vi "Stop Core.vi"(10 "final error code":i32, 11 "Red Pitaya in":refnum<class "Red Pitaya.lvclass">) -> (3 "Red Pitaya out":refnum<class "Red Pitaya.lvclass">)   [LabVIEW 2015, in "Red Pitaya.lvclass"]
doc: "(<B>Filename</B>: Actor Framework.lvlib:Actor.lvclass:Stop Core.vi)\n\nDefines what the actor does before it stops. Use the <B>final error code</B> input to determine whether the actor shut down in response to an error.\n\nBy default, this method does nothing. A descendant class may override it to define behavior, such as shutting down any processes the actor initiated in its override of the Actor Core method."
uses:
  Red Pitaya.lvclass
  Mag Lab Measure/Hardware/Digitizer/Mag Lab Digitizer.lvclass
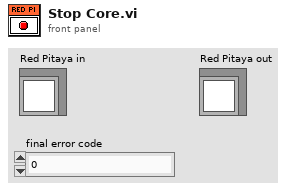
[diagram p1: front panel]
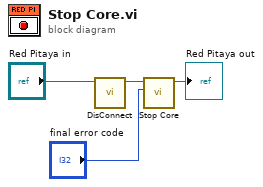
[diagram p0: block diagram]
diagram:
  n1 = call "DisConnect.vi"("Red Pitaya in"="Red Pitaya in") -> ("Red Pitaya out"=w2:refnum<class "Red Pitaya.lvclass">)  [unwired: 9 in, 1 out]
  n2 = call-parent "Stop Core.vi"("final error code"="final error code", "Mag Lab Measure Base in"=w2) -> ("Mag Lab Measure Base out"=→"Red Pitaya out":refnum<class "Red Pitaya.lvclass">)  [unwired: 9 in]
